vi "FTW-SQLite-LibraryFilepath.vi"(8 "error in":errorcluster, 10 "Rediscover library?":bool) -> (0 "error out":errorcluster, 1 "SQLite Version":string, 2 "SQLite Library Filepath":path)   [LabVIEW 2012, in "FTW-SQLite-Connector.lvclass"]
uses:
  FTW-SQLite-Connector.lvclass
panel:
  # "Inputs"
  # "Outputs"
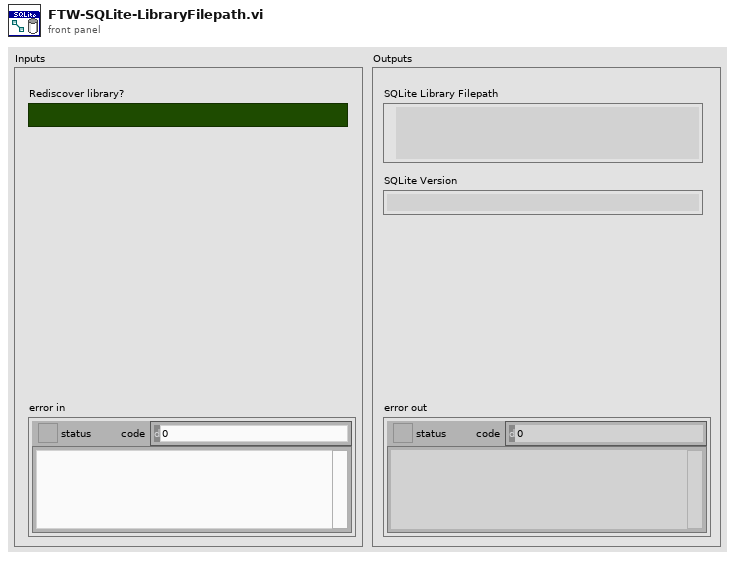
[diagram p1: front panel]
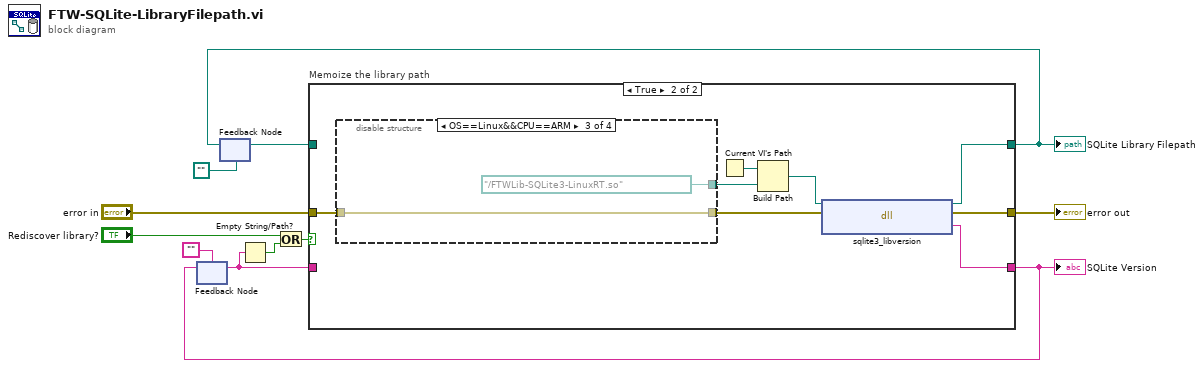
[diagram p0: block diagram]
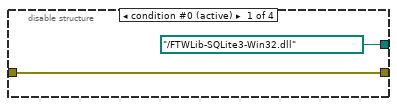
[diagram p3: hidden frame]
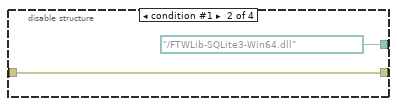
[diagram p4: hidden frame]
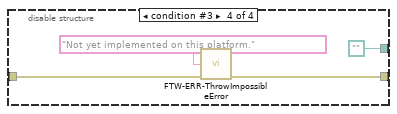
[diagram p5: hidden frame]
diagram:
  n1 = feedback #1("") -> (w4:string)
  n2 = feedback #2(path "") -> (w9:path)
  n3 = Empty String/Path?(string/path=w4) -> (empty?=w3:bool)
  n4 = Or(x="Rediscover library?", y=w3) -> (x .or. y?=w5:bool)
  n5 = case "Memoize the library path" shown="True" w5 {
    tunnel: [w14 w18] -> w8
    tunnel: "error in" -> [w13 w22]
    tunnel: [w12 w19] -> w7
    tunnel: [w13 w17] -> w10
    tunnel: w9 -> [w14 _]
    tunnel: w4 -> [w12 _]
    frame False {
    }
    frame True {
      n6 = disable-structure shown="OS==Linux&&CPU==ARM" {
        disable-tunnel: [path "../FTWLib-SQLite3-Win32.dll" path "../FTWLib-SQLite3-Win64.dll" path "../FTWLib-SQLite3-LinuxRT.so" path ""] -> w20
        disable-tunnel: [w24 w25 w27 w31] -> w15
        disable-tunnel: w22 -> [w24 w25 w27 w32]
        frame condition #0 (active) {
        }
        frame condition #1 {
        }
        frame condition #2 {
        }
        frame condition #3 {
          n7 = call "FTW-ERR-ThrowImpossibleError.vi"("Reason this error should never happen"="Not yet implemented on this platform.", "error in"=w32) -> ("error out"=w31:errorcluster)  [unwired: 13 in]
        }
      }
      n8 = Current VI's Path() -> (path=w21:path)
      n9 = Build Path(base path=w21, name or relative path=w20) -> (appended path=w16:path)
      n10 = dll-call lib="?" fn="sqlite3_libversion"(path in=w16, error in=w15) -> (path out=w18:path, error out=w17:errorcluster, "Return Value"=w19:string)  [unwired: 1 in]
    }
  }
  "error out" <- w10
  "SQLite Library Filepath" <- w8
  "SQLite Version" <- w7
  n11 = feedback-in #1(w7) -> ()
  n12 = feedback-in #2(w8) -> ()
